vi "UI_Color.vi"(0 "State in":T1={"State 1"={"BG"=0, "FG"=0}, "State 0"={"BG"=0, "FG"=0}, "State 2"={"BG"=0, "FG"=0}, "State 3"={"BG"=0, "FG"=0}, "Shortcut Menu"=enum."Do left-click popup"} caption="State", 5 "FP.Title":string, 11 "error in":errorcluster) -> (4 "State out":T1={"State 1"={"BG"=0, "FG"=0}, "State 0"={"BG"=0, "FG"=0}, "State 2"={"BG"=0, "FG"=0}, "State 3"={"BG"=0, "FG"=0}, "Shortcut Menu"=enum."Do left-click popup"} caption="State", 15 "error out":errorcluster)   [LabVIEW 2011, in "Led.xctl"]
doc: "This UI allows colors modification by user during execution."
uses:
  Led.xctl
  State.ctl
  TD_Status.ctl
panel:
  in  "Color 3":u32(colorbox) caption="Error"
  in  "Cancel":bool
  in  "OK Button":bool
  in  "Color 2":u32(colorbox) caption="Connecting"
  in  "Color 1":u32(colorbox) caption="Connected"
  in  "Color 0":u32(colorbox) caption="Disconnected"
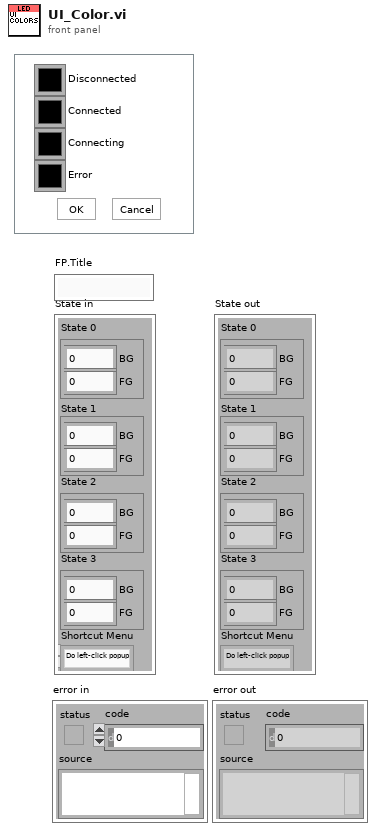
[diagram p1: front panel]
types:
  T1 = typedef "Led.xctl/State.ctl" = cluster{"State 1":cluster{"BG":u32, "FG":u32}, "State 0":cluster{"BG":u32, "FG":u32}, "State 2":cluster{"BG":u32, "FG":u32}, "State 3":cluster{"BG":u32, "FG":u32}, "Shortcut Menu":enum16{"Treat normally", "Do left-click popup"}}
  T2 = typedef "Led.xctl/TD_Status.ctl" = enum16{"Disconnected", "Connected", "Connecting", "Error"}
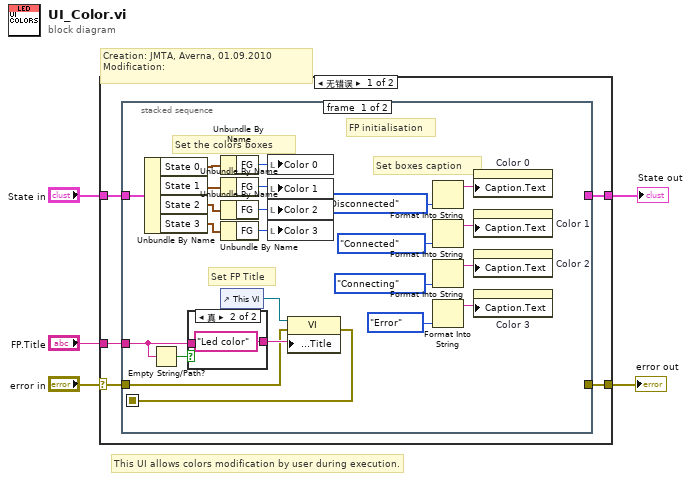
[diagram p0: block diagram]
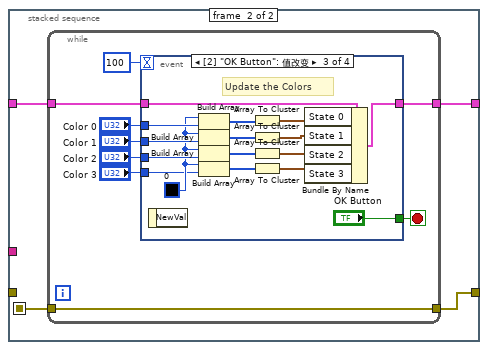
[diagram p3: hidden frame]
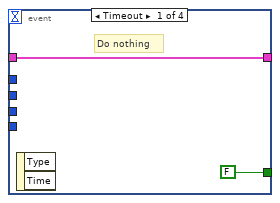
[diagram p4: hidden frame]
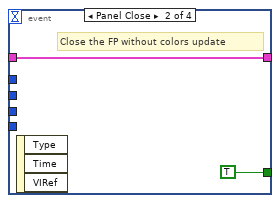
[diagram p5: hidden frame]
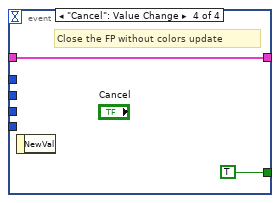
[diagram p6: hidden frame]
diagram:
  # "This UI allows colors modification by user during execution."
  # "Creation: JMTA, Averna, 01.09.2010 \nModification:"
  n1 = case shown="无错误" "error in" {
    selector: "error in" -> [w9 w72]
    tunnel: [w10 w72] -> w4
    tunnel: "State in" -> [w8 w71]
    tunnel: [w7 w71] -> w2
    tunnel: "FP.Title" -> [w6 _]
    frame No Error {
      n2 = stacked-sequence {
        seq-local: [w29 _] -> [_ w36]
        tunnel: [_ w39] -> w10
        tunnel: w9 -> [w30 _]
        tunnel: w8 -> [w28 w38]
        tunnel: [_ w37] -> w7
        tunnel: w6 -> [w15 _]
        frame #0 {
          # "Set FP Title"
          # "Set boxes caption"
          # "Set the colors boxes"
          # "FP initialisation"
          n3 = Unbundle By Name(w28) -> ("State 0"=w27:cluster{"BG":u32, "FG":u32}, "State 1"=w25:cluster{"BG":u32, "FG":u32}, "State 2"=w24:cluster{"BG":u32, "FG":u32}, "State 3"=w23:cluster{"BG":u32, "FG":u32})
          n4 = Empty String/Path?(string/path=w15) -> (empty?=w32:bool)
          n5 = case shown="真" w32 {
            tunnel: [w34 "Led color" ("Label")] -> w31
            tunnel: w15 -> [w34 _]
            frame False {
            }
            frame True {
            }
          }
          n6 = Unbundle By Name(w27) -> ("FG"=w26:u32)
          n7 = Unbundle By Name(w25) -> ("FG"=w22:u32)
          n8 = Unbundle By Name(w24) -> ("FG"=w21:u32)
          n9 = Unbundle By Name(w23) -> ("FG"=w20:u32)
          n10 = control-ref of="This VI"() -> (w33:refnum<vi>)
          n11 = local write "Color 0"(w26) -> ()
          n12 = local write "Color 1"(w22) -> ()
          n13 = local write "Color 2"(w21) -> ()
          n14 = local write "Color 3"(w20) -> ()
          n15 = property class="VI"(reference=w33, error in=w30, "Front Panel.Title"=w31) -> (error out=w29:errorcluster)  [unwired: 1 out]
          n16 = Format Into String(TD_Status."Disconnected" ("Status")) -> (resulting string=w17:string)  [unwired: 3 in, 1 out]
          n17 = Format Into String(TD_Status."Connected" ("Status")) -> (resulting string=w19:string)  [unwired: 3 in, 1 out]
          n18 = Format Into String(TD_Status."Connecting" ("Status")) -> (resulting string=w12:string)  [unwired: 3 in, 1 out]
          n19 = Format Into String(TD_Status."Error" ("Status")) -> (resulting string=w14:string)  [unwired: 3 in, 1 out]
          n20 = property on="Color 0" class="ColBox"("Caption.Text"=w17) -> ()  [unwired: 2 in, 2 out]
          n21 = property on="Color 1" class="ColBox"("Caption.Text"=w19) -> ()  [unwired: 2 in, 2 out]
          n22 = property on="Color 2" class="ColBox"("Caption.Text"=w12) -> ()  [unwired: 2 in, 2 out]
          n23 = property on="Color 3" class="ColBox"("Caption.Text"=w14) -> ()  [unwired: 2 in, 2 out]
        }
        frame #1 {
          n24 = while {
            tunnel: [w47] -> w39
            tunnel: w36 -> [w47]
            tunnel: w38 -> [w45]
            tunnel: [w44] -> w37
            stop <- w46 stop-if-true
            n25 = event shown="[2] \"OK Button\": 值改变" {
              selector: _ -> [_ _ _ _]
              dyn-events: _ -> [_ _ _ _]
              timeout: 100 -> [_ _ _ _]
              tunnel: [FALSE ("OK Button") TRUE ("OK Button") "OK Button" TRUE ("OK Button")] -> w46
              tunnel: w45 -> [w49 w51 w66 w69]
              tunnel: [w49 w51 w53 w69] -> w44
              tunnel: "Color 0" -> [_ _ w58 _]
              tunnel: "Color 1" -> [_ _ w57 _]
              tunnel: "Color 2" -> [_ _ w56 _]
              tunnel: "Color 3" -> [_ _ w54 _]
              event Timeout {
                # "Do nothing"
                n26 = event-data() -> ()  [unwired: 1 in, 2 out]
              }
              event Panel Close {
                # "Close the FP without colors update"
                n27 = event-data() -> ()  [unwired: 1 in, 3 out]
              }
              event "OK Button": Value Change {
                w55 = u32 0
                # "Update the Colors"
                n28 = event-data() -> ()  [unwired: 1 in, 1 out]
                n29 = Build Array(w55, w58) -> (w67:u32[])
                n30 = Build Array(w55, w57) -> (w62:u32[])
                n31 = Build Array(w55, w56) -> (w64:u32[])
                n32 = Build Array(w55, w54) -> (w60:u32[])
                n33 = Array To Cluster(array=w67) -> (cluster=w65:cluster{"[0]":u32, "[1]":u32})
                n34 = Array To Cluster(array=w62) -> (cluster=w61:cluster{"[0]":u32, "[1]":u32})
                n35 = Array To Cluster(array=w64) -> (cluster=w63:cluster{"[0]":u32, "[1]":u32})
                n36 = Array To Cluster(array=w60) -> (cluster=w59:cluster{"[0]":u32, "[1]":u32})
                n37 = Bundle By Name(cluster=w66, "State 0"=w65, "State 1"=w61, "State 2"=w63, "State 3"=w59) -> (w53:T1)
              }
              event "Cancel": Value Change {
                # "Close the FP without colors update"
                n38 = event-data() -> ()  [unwired: 1 in, 1 out]
              }
            }
          }
        }
      }
    }
    frame Error {
    }
  }
  "error out" <- w4
  "State out" <- w2
